vi "getParAndArgChkRes.vi"(8 "error in":errorcluster, 9 "func":string, 10 "arg":string, 11 "Tree Refnum in":refnum<vi>) -> (0 "error out":errorcluster, 1 "Check result":string="√", 2 "par":string, 3 "Tree Refnum out":refnum<vi>)   [LabVIEW 2010]
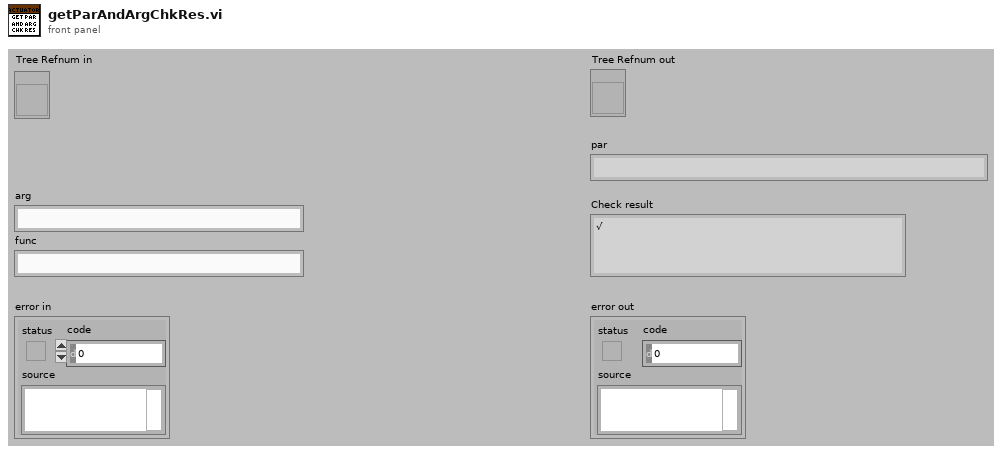
[diagram p1: front panel]
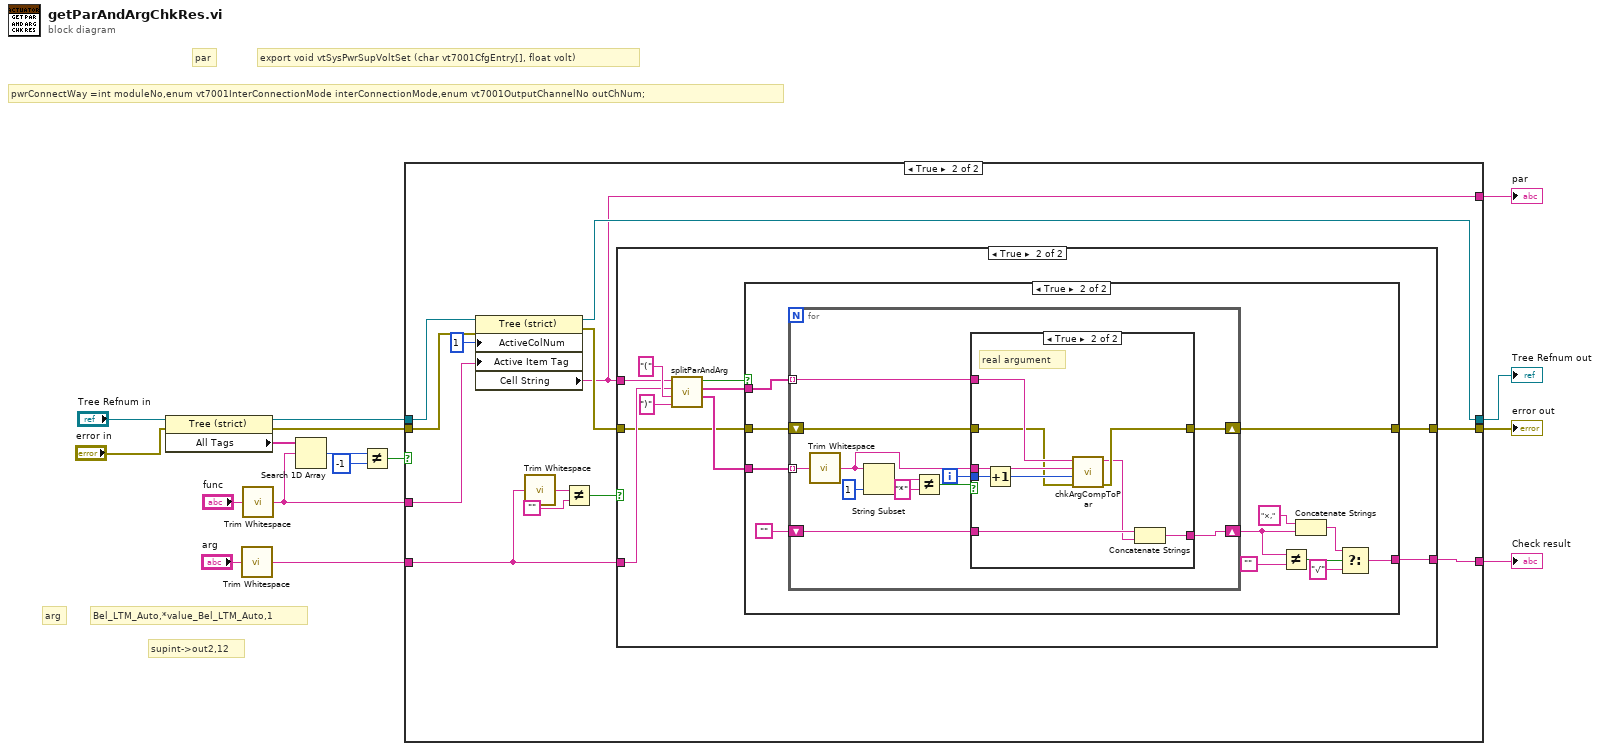
[diagram p0: block diagram]
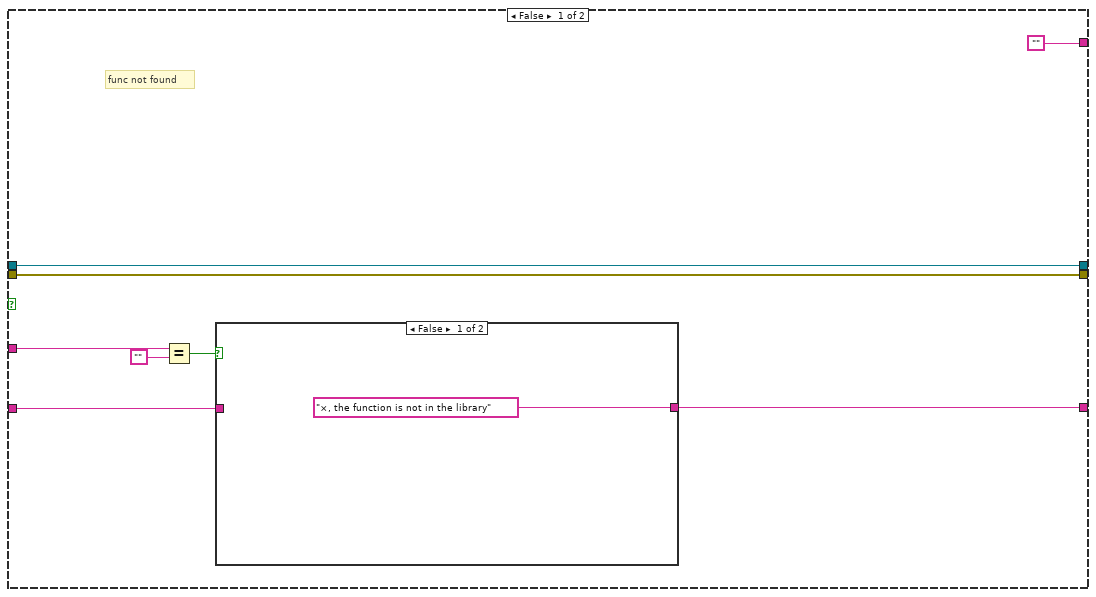
[diagram p2: hidden frame]
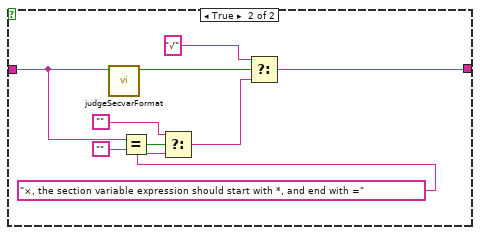
[diagram p3: hidden frame]
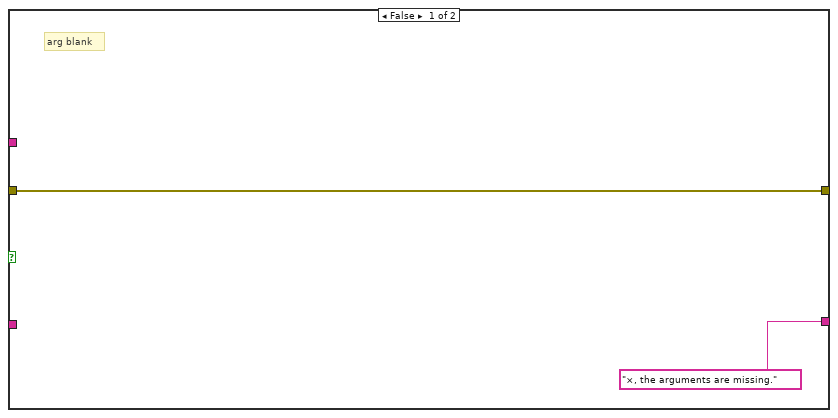
[diagram p4: hidden frame]
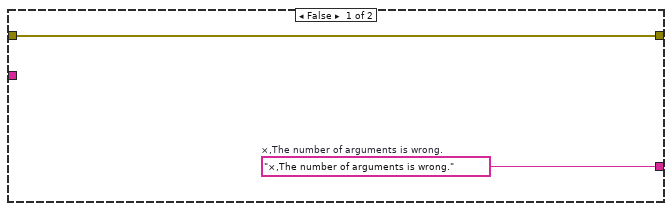
[diagram p5: hidden frame]
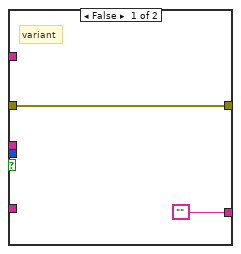
[diagram p6: hidden frame]
diagram:
  # "pwrConnectWay =int moduleNo,enum vt7001InterConnectionMode interConnectionMode,enum vt7001OutputChannelNo outChNum;"
  # "arg"
  # "par"
  # "Bel_LTM_Auto,*value_Bel_LTM_Auto,1"
  # "supint->out2,12"
  # "export void vtSysPwrSupVoltSet (char vt7001CfgEntry[], float volt)"
  n1 = property on="Property Node" class="Tree (strict)"(reference="Tree Refnum in", error in="error in") -> (reference out=w9:refnum<vi>, error out=w10:errorcluster, "All Tags"=w13:string[])
  n2 = call <vilib>:"Trim Whitespace.vi"("string"="arg") -> ("trimmed string"=w5:string)  [unwired: 1 in]
  n3 = call <vilib>:"Trim Whitespace.vi"("string"="func") -> ("trimmed string"=w6:string)  [unwired: 1 in]
  n4 = Search 1D Array(1D array=w13, element=w6) -> (index of element=w12:i32)  [unwired: 1 in]
  n5 = Not Equal?(x=w12, y=-1) -> (x != y?=w16:bool)
  n6 = case shown="True" w16 {
    tunnel: w5 -> [w21 w42]
    tunnel: w10 -> [w18 w40]
    tunnel: [w20 w47] -> w15
    tunnel: [w18 w46] -> w14
    tunnel: w9 -> [w19 w38]
    tunnel: [w19 w36] -> w8
    tunnel: w6 -> [w24 w39]
    tunnel: ["" w35] -> w1
    frame False {
      # "func not found"
      n7 = Equal?(x=w24, y="") -> (x = y?=w22:bool)
      n8 = case shown="False" w22 {
        tunnel: w21 -> [_ w27]
        tunnel: ["×, the function is not in the library" w33] -> w20
        frame False {
        }
        frame True {
          n9 = call "judgeSecvarFormat.vi"("section variable"=w27) -> ("correct format?"=w28:bool)  [unwired: 10 in]
          n10 = Equal?(x=w27, y="") -> (x = y?=w32:bool)
          n11 = Select(t="", s=w32, f="×, the section variable expression should start with *, and end with =" ("Value")) -> (s? t:f=w26:string)
          n12 = Select(t="√", s=w28, f=w26) -> (s? t:f=w33:string)
        }
      }
    }
    frame True {
      n13 = property class="Tree (strict)"(reference=w38, error in=w40, "ActiveColNum"=1 ("Active Cell:Active Column Number"), "Active Item Tag"=w39) -> (reference out=w36:refnum<vi>, error out=w37:errorcluster, "Cell String"=w35:string)
      n14 = call <vilib>:"Trim Whitespace.vi"("string"=w42) -> ("trimmed string"=w45:string)  [unwired: 1 in]
      n15 = Not Equal?(x=w45, y="") -> (x != y?=w43:bool)
      n16 = case shown="True" w43 {
        tunnel: w35 -> [_ w55]
        tunnel: w42 -> [_ w54]
        tunnel: w37 -> [w49 w50]
        tunnel: ["×, the arguments are missing." w59] -> w47
        tunnel: [w49 w58] -> w46
        frame False {
          # "arg blank"
        }
        frame True {
          n17 = call "splitParAndArg.vi"("paraEndMark"=")" ("regular expression"), "paraStartMark"="(" ("regular expression"), "allArguments"=w54, "allParameters"=w55) -> ("argArray"=w52:string[], "paraArray"=w53:string[], "sameNum?"=w51:bool)  [unwired: 5 in]
          n18 = case shown="True" w51 {
            tunnel: w53 -> [_ w73]
            tunnel: w52 -> [_ w72]
            tunnel: [w61 w67] -> w59
            tunnel: w50 -> [w60 w66]
            tunnel: [w60 w65] -> w58
            frame False {
              w61 = "×,The number of arguments is wrong."  # ×,The number of arguments is wrong.
            }
            frame True {
              n19 = for {
                tunnel: w73 -> [w85] mode=indexing
                tunnel: w72 -> [w75] mode=indexing
                shift-right: [w83] -> w63
                shift-left: "" -> [w84]
                shift-right: [w81] -> w65
                shift-left: w66 -> [w82]
                i -> [w76]
                n20 = call <vilib>:"Trim Whitespace.vi"("string"=w75) -> ("trimmed string"=w74:string)  [unwired: 1 in]
                n21 = String Subset(string=w74, length (rest)=1 ("length (rest)")) -> (substring=w79:string)  [unwired: 1 in]
                n22 = Not Equal?(x=w79, y="*") -> (x != y?=w77:bool)
                n23 = case shown="True" w77 {
                  tunnel: w85 -> [_ w93]
                  tunnel: w84 -> [_ w96]
                  tunnel: ["" w95] -> w83
                  tunnel: w82 -> [w86 w90]
                  tunnel: [w86 w89] -> w81
                  tunnel: w76 -> [_ w92]
                  tunnel: w74 -> [_ w94]
                  frame False {
                    # "variant"
                  }
                  frame True {
                    # "real argument"
                    n24 = Increment(x=w92) -> (x+1=w91:i32)
                    n25 = call "chkArgCompToPar.vi"("error in"=w90, "argSN"=w91, "arg"=w94, "par"=w93) -> ("error out"=w89:errorcluster, "judgement"=w88:string)  [unwired: 6 in]
                    n26 = Concatenate Strings(w96, w88) -> (w95:string)
                  }
                }
              }
              n27 = Not Equal?(x=w63, y="") -> (x != y?=w69:bool)
              n28 = Concatenate Strings("×,", w63) -> (w62:string)
              n29 = Select(t=w62, s=w69, f="√") -> (s? t:f=w67:string)
            }
          }
        }
      }
    }
  }
  "Check result" <- w15
  "error out" <- w14
  "Tree Refnum out" <- w8
  "par" <- w1
